vi "Getsettings.vi"(5 "PllCntrl":T1={"PLL PWR"=3, "MUX out"=0, "Phase"=1, "Low Noise"=TRUE, "REF X2"=FALSE, "Mute till LD"=TRUE, "Icp"=15, "Band Sel Div"=100, "REF Divide"=5, "Reference(MHz)"=10.0} {"Icp" scale=0.0..15.0; "MUX out" items=["3-State", "GND", "Vcc", "Analog LD", "Digital LD", "REF / R", "RF / N"]; "PLL PWR" scale=0.0..3.0}, 8 "Step Size  (MHz)":dbl=0.001, 10 "Freq (MHz)":dbl=3001.0 format="%#_7g") -> (0 "Modulus":i32, 1 "INT":i16, 2 "FRAC":i32, 3 "RF Divider":i32, 7 "Pfd (MHz)":dbl=10.0)   [LabVIEW 2013]
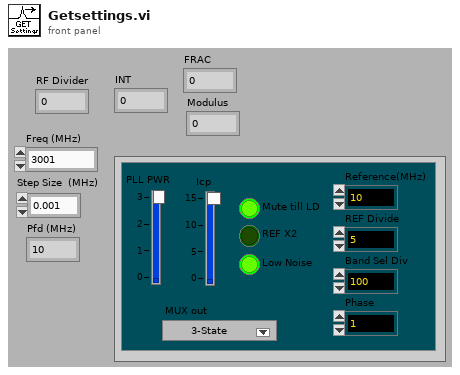
[diagram p1: front panel]
types:
  T1 = cluster{"PLL PWR":i8, "MUX out":u16, "Phase":i16, "Low Noise":bool, "REF X2":bool, "Mute till LD":bool, "Icp":i32, "Band Sel Div":i32, "REF Divide":i16, "Reference(MHz)":dbl}
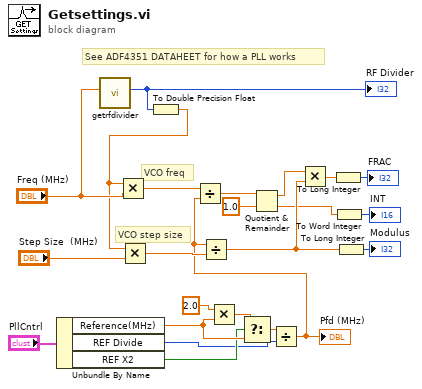
[diagram p0: block diagram]
diagram:
  # "VCO step size"
  # "VCO freq"
  # "See ADF4351 DATAHEET for how a PLL works"
  n1 = Unbundle By Name("PllCntrl") -> ("Reference(MHz)"=w5:dbl, "REF Divide"=w3:i16, "REF X2"=w4:bool)
  n2 = call "getrfdivider.vi"("Frequency (MHz)"="Freq (MHz)") -> ("RF Divider"=w20:i32)  [unwired: 10 in]
  "RF Divider" <- w20
  n3 = To Double Precision Float(number=w20) -> (double precision float=w19:dbl)
  n4 = Multiply(x=w19, y="Freq (MHz)") -> (x*y=w18:dbl)
  n5 = Multiply(x=w19, y="Step Size  (MHz)") -> (x*y=w23:dbl)
  n6 = Multiply(x=2.0, y=w5) -> (x*y=w7:dbl)
  n7 = Select(t=w7, s=w4, f=w5) -> (s? t:f=w8:dbl)
  n8 = Divide(x=w8, y=w3) -> (x/y=w1:dbl)
  "Pfd (MHz)" <- w1
  n9 = Divide(x=w18, y=w1) -> (x/y=w17:dbl)
  n10 = Divide(x=w1, y=w23) -> (x/y=w12:dbl)
  n11 = Quotient & Remainder(x=w17, y=1.0) -> (x-y*floor(x/y)=w15:dbl, floor(x/y)=w10:dbl)
  n12 = Multiply(x=w15, y=w12) -> (x*y=w9:dbl)
  n13 = To Long Integer(number=w9) -> (32bit integer=→"FRAC":i32)
  n14 = To Word Integer(number=w10) -> (16bit integer=→"INT":i16)
  n15 = To Long Integer(number=w12) -> (32bit integer=→"Modulus":i32)
